vi "Validate Name.vi"(8 "error in (no error)":errorcluster, 11 "Name":string) -> (0 "error out":errorcluster, 3 "Valid Name":bool)   [LabVIEW 2020, in "Metrics.lvlib" / "Metric.lvclass"]
uses:
  Metric.lvclass
  <vilib>/regexp/Match Regular Expression.xnode
  Metric.lvclass/Metric.ctl
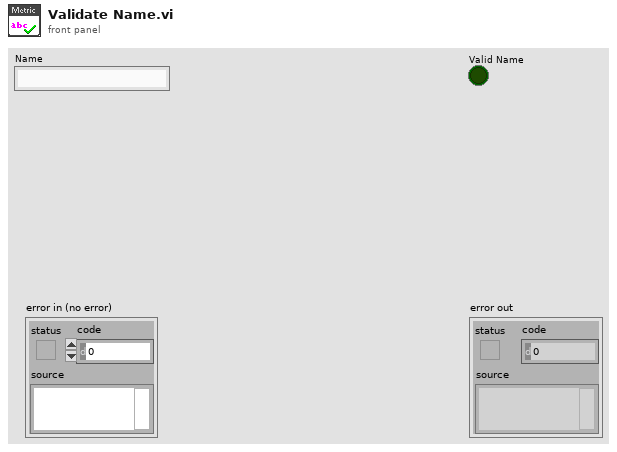
[diagram p1: front panel]
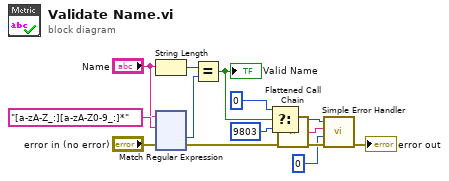
[diagram p0: block diagram]
diagram:
  n1 = String Length(string="Name") -> (length=w10:i32)
  n2 = xnode "Match Regular Expression"("input string"="Name", "regular expression"="[a-zA-Z_:][a-zA-Z0-9_:]*", "error in"="error in (no error)") -> ("offset past match"=w11:i32, "error out"=w3:errorcluster)  [unwired: 3 in, 3 out]
  n3 = Equal?(x=w10, y=w11) -> (x = y?=w9:bool)
  "Valid Name" <- w9
  n4 = Select(t=0 ("error code (no error:0)"), s=w9, f=9803 ("error code (no error:0)")) -> (s? t:f=w4:i32)
  n5 = call "Flattened Call Chain.vi"() -> ("Flattened Call Chain"=w2:string)  [unwired: 5 in]
  n6 = call <vilib>:"Simple Error Handler.vi"("error code (no error:0)"=w4, "error source (\" \")"=w2, "type of dialog (OK msg:1)"=0 ("error code (no error:0)"), "error in (no error)"=w3) -> ("error out"=→"error out":errorcluster)  [unwired: 1 in, 4 out]
